vi "Pressurize.vi"(8 "error in (no error)":errorcluster, 11 "cetoni in":refnum<class "cetoni.lvclass">) -> (0 "error out":errorcluster, 3 "cetoni out":refnum<class "cetoni.lvclass">)   [LabVIEW 2018, in "cetoni.lvlib" / "cetoni.lvclass"]
uses:
  cetoni.lvclass
  <userlib>/QmixLib/QmixLib.lvlib
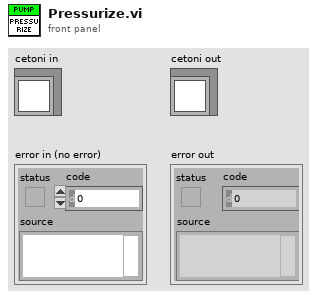
[diagram p1: front panel]
types:
  T1 = enum16{"LOW_PRESSURE_VALVE", "BALL_VALVE", "QMIX_VALVE"}
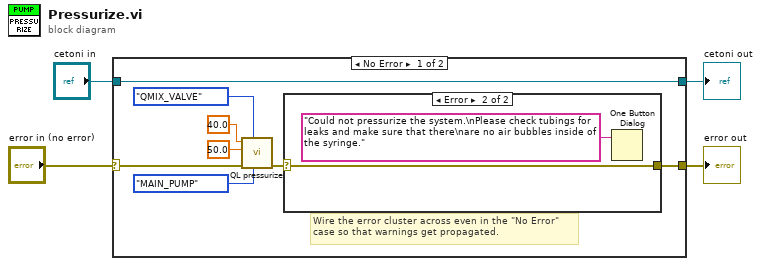
[diagram p0: block diagram]
diagram:
  n1 = case shown="No Error" "error in (no error)" {
    selector: "error in (no error)" -> [w11 w17]
    tunnel: [w5 w17] -> w3
    tunnel: [w12 w16] -> w1
    tunnel: "cetoni in" -> [w12 w16]
    frame No Error {
      # "Wire the error cluster across even in the \"No Error\"\ncase so that warnings get propagated."
      n2 = call <userlib>:"QL pressurize.vi"("pump"=enum16{"MAIN_PUMP"}."MAIN_PUMP", "valve"=T1."QMIX_VALVE", "error in (no error)"=w11, "flow_rate_uL_s"=50.0, "max_pressure"=40.0) -> ("error out"=w6:errorcluster)  [unwired: 6 in]
      n3 = case shown="Error" w6 {
        selector: w6 -> [w13 w15]
        tunnel: [w13 w15] -> w5
        frame No Error {
        }
        frame Error {
          n4 = One Button Dialog(message="Could not pressurize the system.\nPlease check tubings for leaks and make sure that there\nare no air bubbles inside of the syringe.") -> ()  [unwired: 1 in, 1 out]
        }
      }
    }
    frame Error {
    }
  }
  "error out" <- w3
  "cetoni out" <- w1
